vi "Read String.vi"(7 "key":string, 8 "error in (no error)":errorcluster, 9 "default value":string, 11 "Configuration File In":refnum<class "Configuration File.lvclass">) -> (0 "error out":errorcluster, 1 "value":string, 3 "Configuration File Out":refnum<class "Configuration File.lvclass">)   [LabVIEW 2020, in "Configuration File.lvclass"]
doc: "High-level function for reading configuration file data from process class. If the specified key is not present, it is added with the configured default value."
uses:
  Configuration File.lvclass
  <vilib>/Utility/config.llb/Read Key (String).vi
  <vilib>/Utility/config.llb/Write Key (String).vi
  <vilib>/Utility/config.llb/NI_LVConfig.lvlib
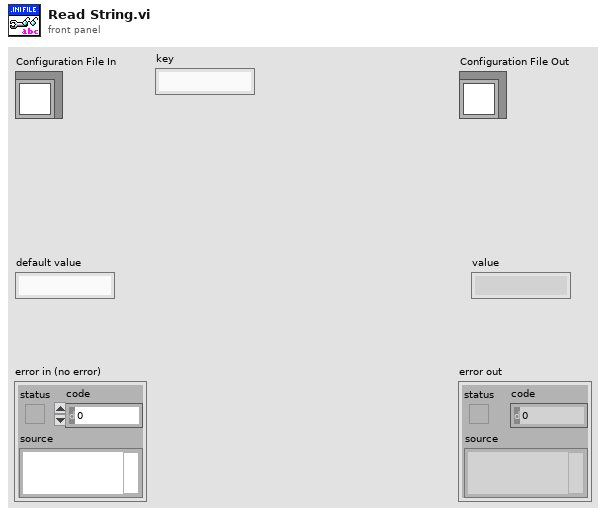
[diagram p1: front panel]
types:
  T1 = typedef "NI_LVConfig.lvlib/Config Data RefNum.ctl" = refnum<k1>
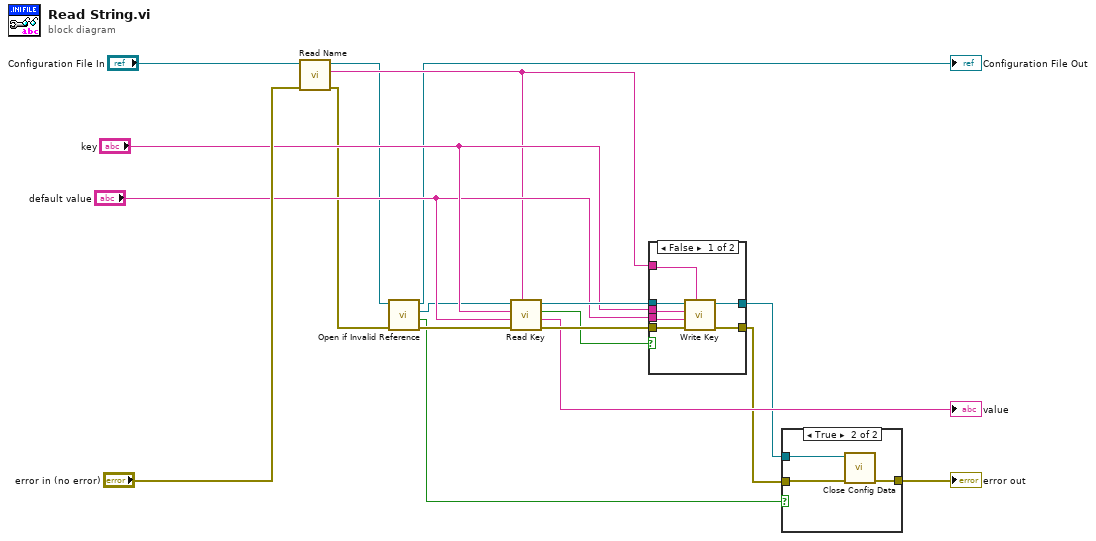
[diagram p0: block diagram]
diagram:
  n1 = call-dynamic "Read Name.vi"("error in (no error)"="error in (no error)", "Configuration File In"="Configuration File In") -> ("error out"=w8:errorcluster, "Name"=w12:string, "Configuration File Out"=w10:refnum<class "Configuration File.lvclass">)  [unwired: 6 in, 1 out]
  n2 = call "Open if Invalid Reference.vi"("error in (no error)"=w8, "Configuration File In"=w10) -> ("error out"=w7:errorcluster, "File opened?"=w2:bool, "refnum out"=w6:T1, "Configuration File Out"=→"Configuration File Out":refnum<class "Configuration File.lvclass">)  [unwired: 6 in]
  n3 = call-poly <vilib>:"Read Key.vi"("section"=w12, "error in (no error)"=w7, "default value"="default value", "key"="key", "refnum"=w6) -> ("error out"=w16:errorcluster, "value"=→"value":string, "found?"=w15:bool, "refnum out"=w17:T1)  [unwired: 3 in]
  n4 = case shown="False" w15 {
    tunnel: w17 -> [w25 w27]
    tunnel: w16 -> [w24 w26]
    tunnel: [w23 w27] -> w3
    tunnel: [w22 w26] -> w5
    tunnel: "key" -> [w21 _]
    tunnel: "default value" -> [w20 _]
    tunnel: w12 -> [w19 _]
    frame False {
      n5 = call-poly <vilib>:"Write Key.vi"("section"=w19, "error in (no error)"=w24, "value"=w20, "key"=w21, "refnum"=w25) -> ("error out"=w22:errorcluster, "refnum out"=w23:T1)  [unwired: 4 in, 1 out]
    }
    frame True {
    }
  }
  n6 = case shown="True" w2 {
    tunnel: w3 -> [_ w31]
    tunnel: w5 -> [w28 w30]
    tunnel: [w28 w29] -> w4
    frame False {
    }
    frame True {
      n7 = call <vilib>:"Close Config Data.vi"("error in (no error)"=w30, "refnum"=w31) -> ("error out"=w29:errorcluster)  [unwired: 8 in, 1 out]
    }
  }
  "error out" <- w4
